vi "SCPI Read Program Data.vi"(8 "error in (no error)":errorcluster, 10 "Step":u16, 11 "VISA resource name":refnum<visa-resource-name>) -> (0 "error out":errorcluster, 1 "Set Current":dbl format="%.2g", 2 "Set Voltage":dbl format="%.2g", 3 "VISA resource name out":refnum<visa-resource-name>, 4 "MIN":dbl format="%.2g", 5 "Elapse Time":u16)   [LabVIEW 2021, in "BK Precision 169XB.lvlib"]
doc: "Returns the actual voltage level and actual current level for a desired channel."
uses:
  BK Precision 169XB.lvlib
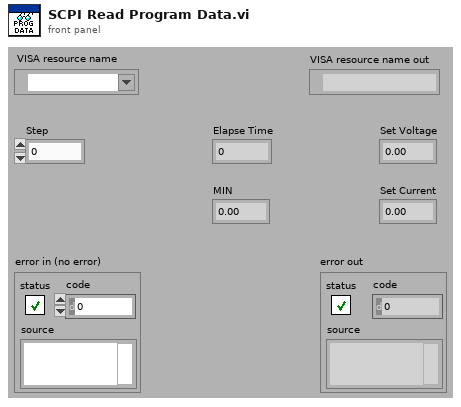
[diagram p1: front panel]
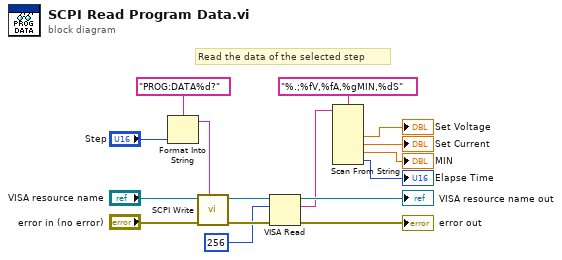
[diagram p0: block diagram]
diagram:
  # "Read the data of the selected step"
  n1 = Format Into String(format string="PROG:DATA%d?" ("Input String"), "Step") -> (resulting string=w3:string)  [unwired: 2 in, 1 out]
  n2 = call "SCPI Write.vi"("Input String"=w3, "error in (no error)"="error in (no error)", "VISA resource name"="VISA resource name") -> ("error out"=w15:errorcluster, "VISA resource name out"=w14:refnum<visa-resource-name>)  [unwired: 7 in]
  n3 = VISA Read(VISA resource name=w14, byte count=u32 256, error in (no error)=w15) -> (VISA resource name out=→"VISA resource name out":refnum<visa-resource-name>, read buffer=w10:string, error out=→"error out":errorcluster)  [unwired: 1 out]
  n4 = Scan From String(format string="%.;%fV,%fA,%gMIN,%dS", input string=w10) -> (output 1=→"Set Voltage":dbl, output 2=→"Set Current":dbl, output 3=→"MIN":dbl, output 4=→"Elapse Time":u16)  [unwired: 6 in, 3 out]
